vi "SP_Breakdown_Analysis.vi"() -> ()   [LabVIEW 2017]
uses:
  <vilib>/addons/database/Connection.llb/DB Tools Open Connec (Path).vi
  Globle/Login Data.vi
  <vilib>/addons/database/NI_Database_API.lvlib
panel:
  out "Elements Found out":string[](array[string])
  in  "Cancel Button - Archive":bool
  out "stackholder":string
  out "Role Id":string
  in  "Get Rport 2":bool
  in  "Download 2":bool
  out "Array":string[][](array[string])
  out "index of element":i32
  in  "Station":string(combo)
  out "error out":errorcluster
  in  "error in (no error)":errorcluster
  in  "Shift":string(combo)
  in  "Tab Control":enum32{"Statistical", "Graphical"}(tab)
  out "Table":string[][](table)
  out "Run-Time Status":cluster{dbl[], dbl[]}(graph)
  in  "To":timestamp format="%<%Y-%m-%d>T"
  in  "From":timestamp format="%<%Y-%m-%d>T"
  in  "Stakeholder":string(combo)
  # "Breakdown Analysis Report"
  # "Designed And Developed By - Infinity Automation Systems Pvt. Ltd."
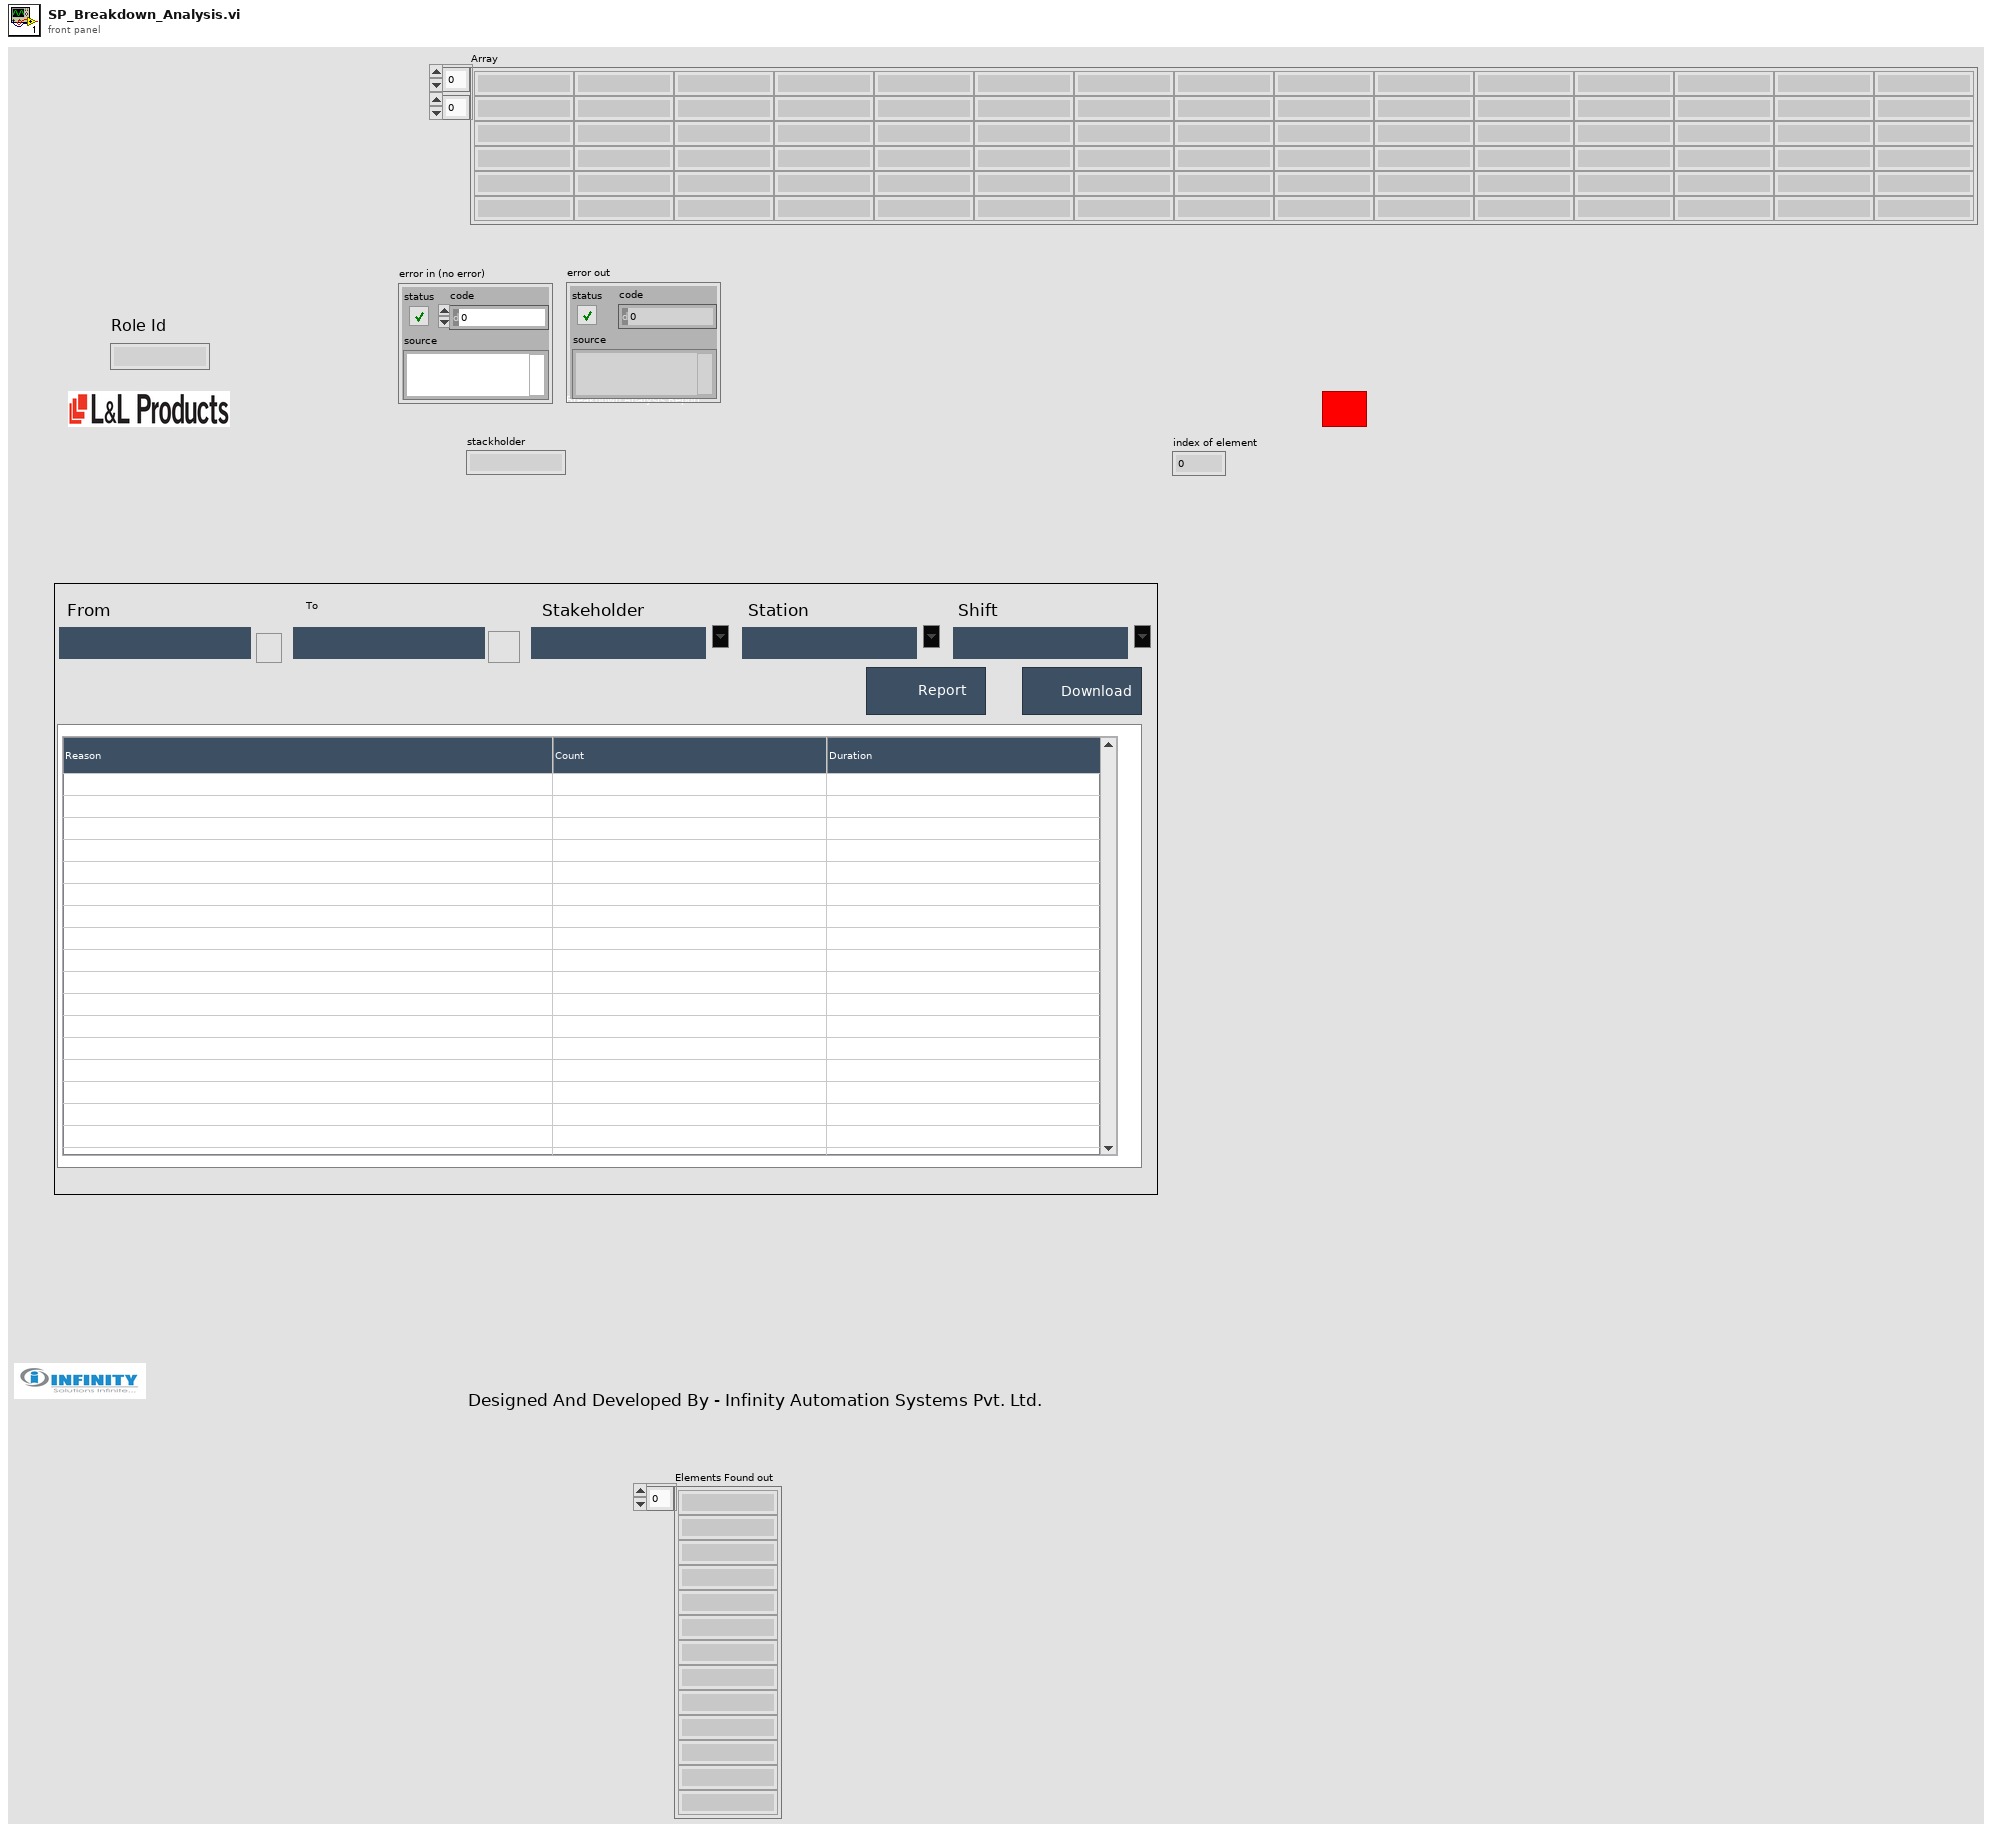
[diagram p1: front panel]
types:
  T1 = typedef "NI_Database_API.lvlib/Conn ObjectReference.ctl" = refnum<k1>
  T2 = enum32{"invalid app kind", "Development System", "Run Time System", "Student Edition", "Embedded LabVIEW", "Evaluation", "Custom"}
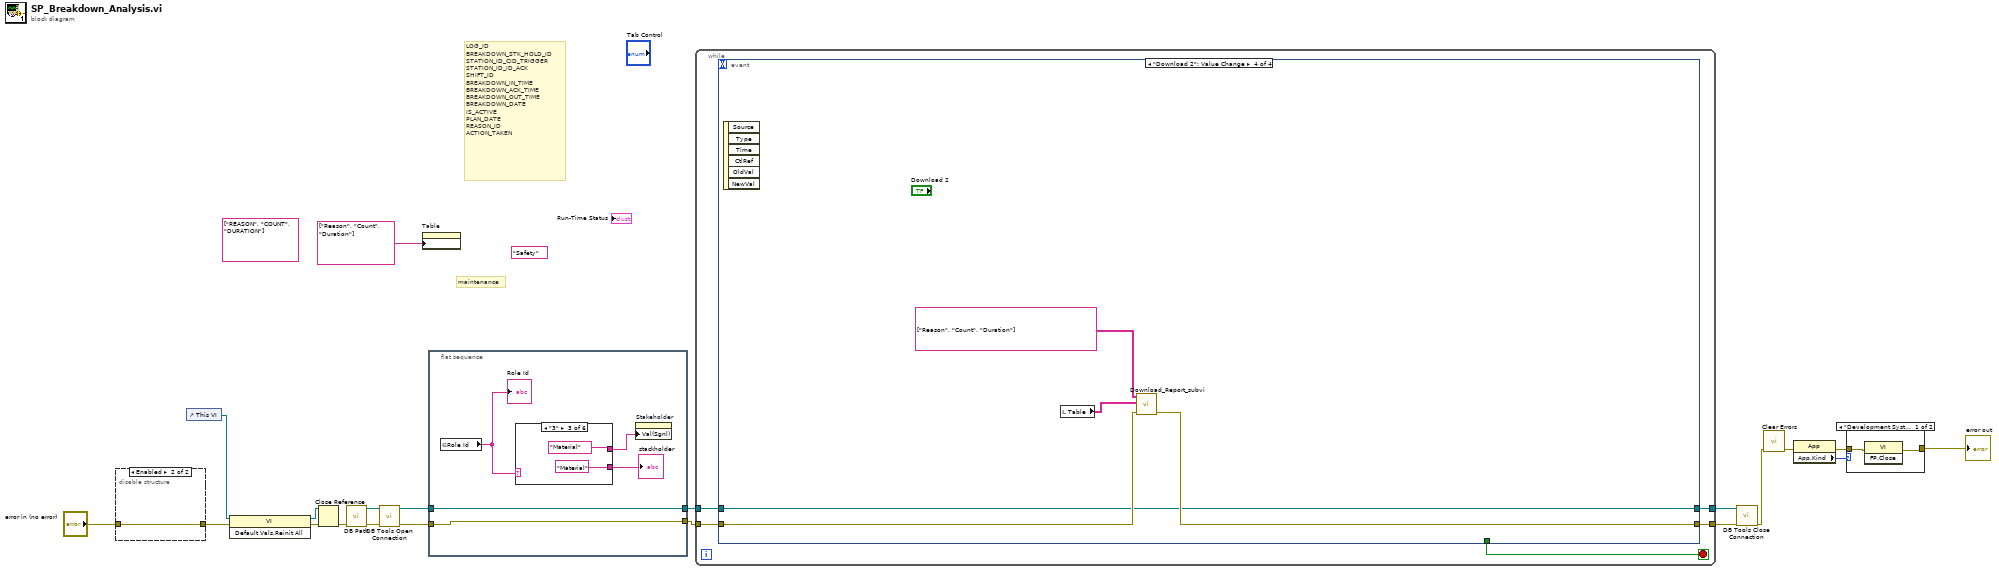
[diagram p0: block diagram]
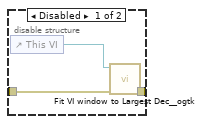
[diagram p2: hidden frame]
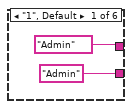
[diagram p3: hidden frame]
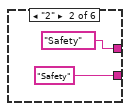
[diagram p4: hidden frame]
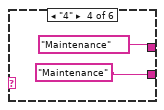
[diagram p5: hidden frame]
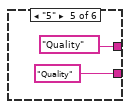
[diagram p6: hidden frame]
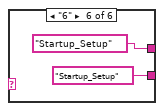
[diagram p7: hidden frame]
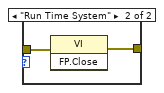
[diagram p8: hidden frame]
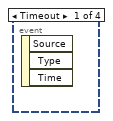
[diagram p9: hidden frame]
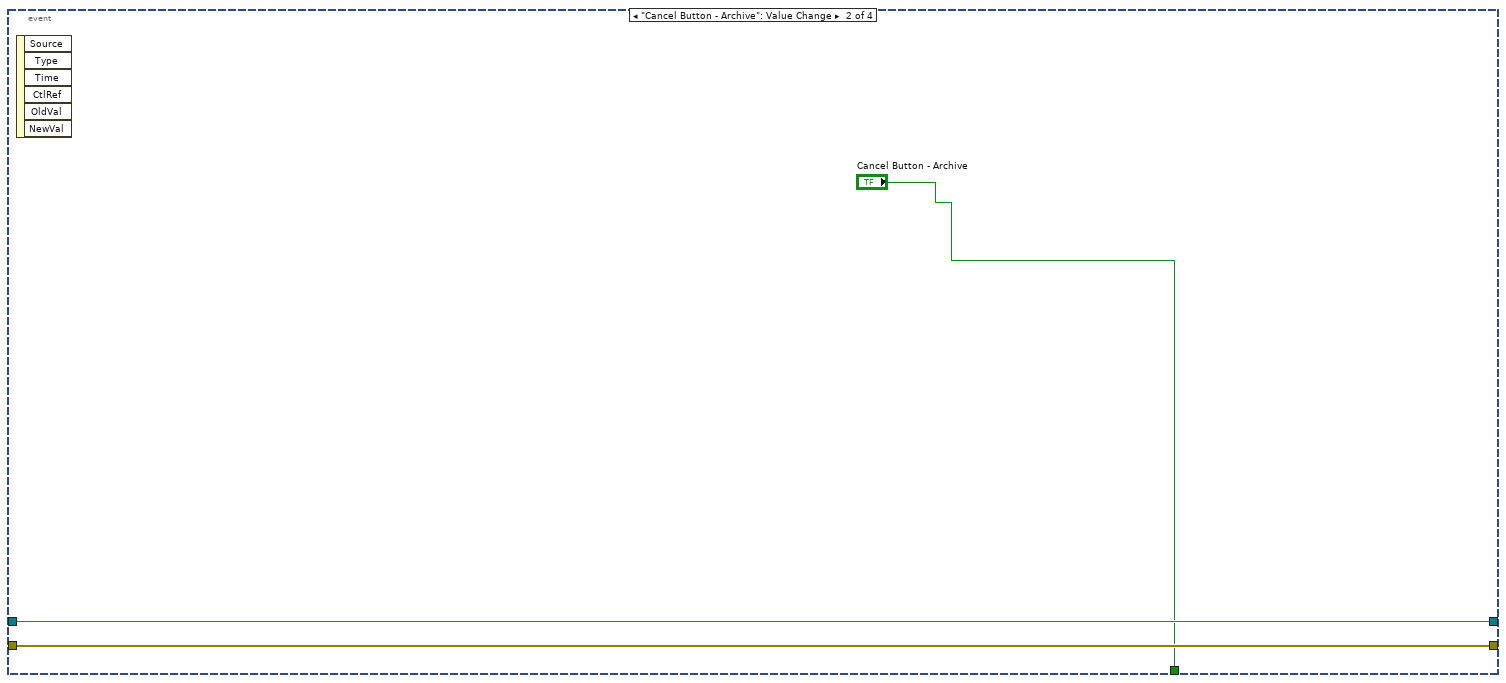
[diagram p10: hidden frame]
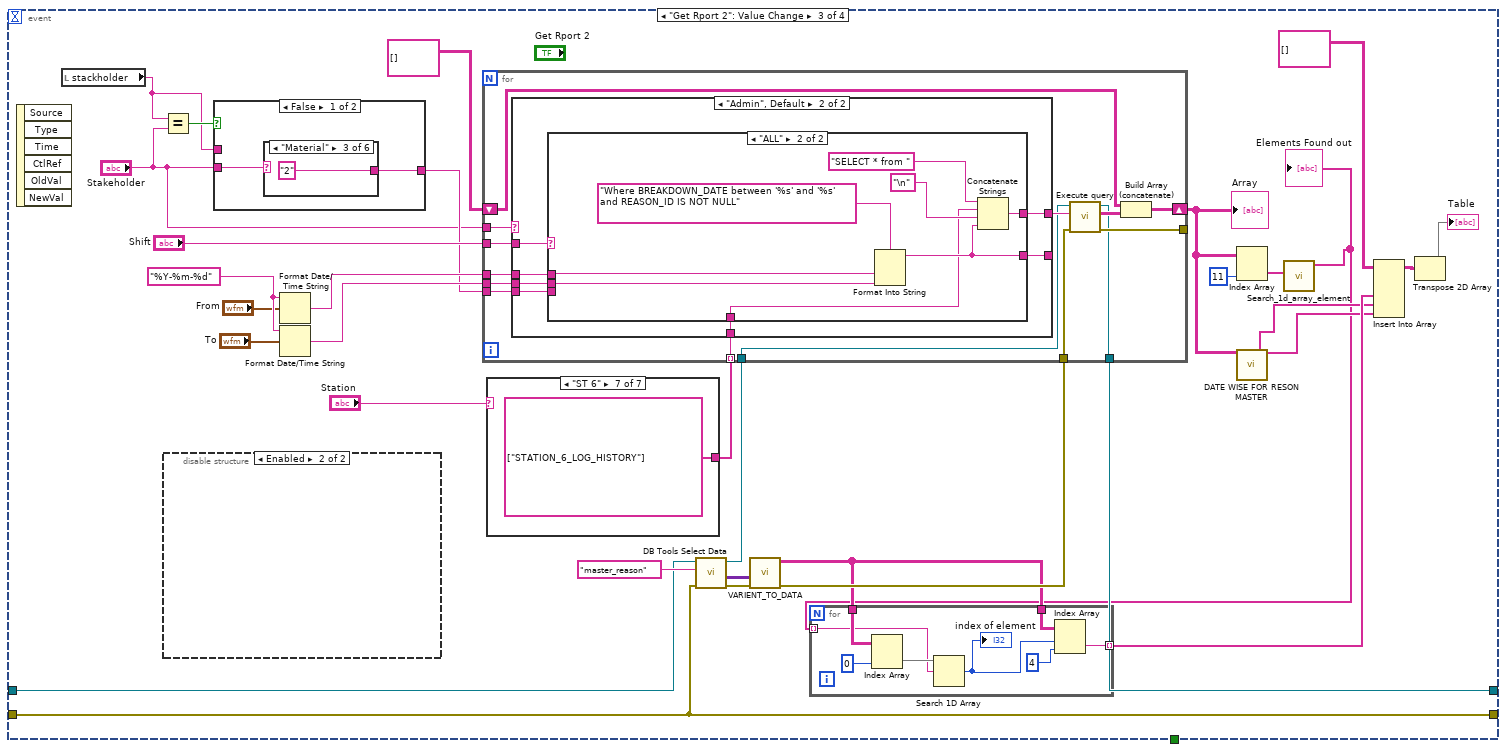
[diagram p11: hidden frame]
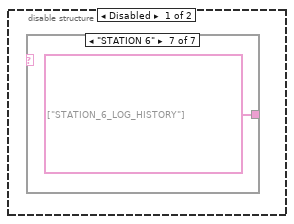
[diagram p12: hidden frame]
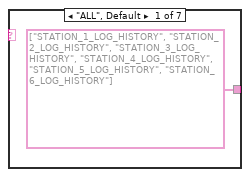
[diagram p13: hidden frame]
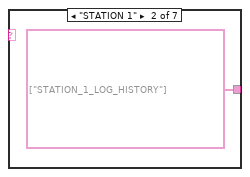
[diagram p14: hidden frame]
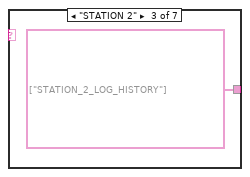
[diagram p15: hidden frame]
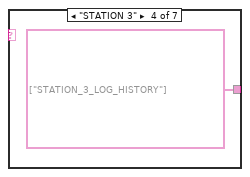
[diagram p16: hidden frame]
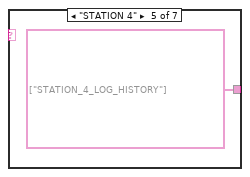
[diagram p17: hidden frame]
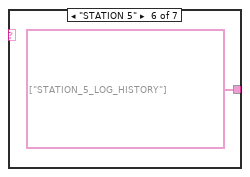
[diagram p18: hidden frame]
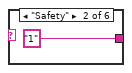
[diagram p20: hidden frame]
diagram:
  (unwired) string[] ["REASON", "COUNT", "DURATION"] ("Column Header Strings[]")
  (unwired) "Safety" ("Stakeholder")
  # "maintenance"
  # "LOG_ID\nBREAKDOWN_STK_HOLD_ID\nSTATION_ID_CID_TRIGGER\nSTATION_ID_ID_ACK\nSHIFT_ID\nBREAKDOWN_IN_TIME\nBREAKDOWN_ACK_TIME\nBREAKDOWN_OUT_TIME\nBREAKDOWN_DATE\nIS_ACTIVE\nPLAN_DATE\nREASON_ID\nACTION_TAKEN"
  n1 = disable-structure shown="Enabled" {
    disable-tunnel: "error in (no error)" -> [w23 w24]
    disable-tunnel: [w22 w24] -> w10
    frame Disabled {
      n2 = control-ref of="This VI"() -> (w21:refnum<vi>)
      n3 = call <userlib>:"Fit VI window to Largest Dec__ogtk.vi"("error in (no error)"=w23, "VI Ref (calling VI)"=w21) -> ("error out"=w22:errorcluster)  [unwired: 4 in, 1 out]
    }
    frame Enabled {
    }
  }
  n4 = control-ref of="This VI"() -> (w20:refnum<vi>)
  n5 = invoke class="VI" method="Default Vals.Reinit All"(reference=w20, error in=w10) -> (reference out=w18:refnum<vi>, error out=w19:errorcluster)  [unwired: 1 in, 1 out]
  n6 = Close Reference(reference=w18, error in (no error)=w19) -> (error out=w17:errorcluster)
  n7 = call "DB Path.vi"("error in"=w17) -> ("error out"=w16:errorcluster, "DB Path"=w15:path)  [unwired: 9 in]
  n8 = call-poly <vilib>:"DB Tools Open Connection.vi"("error in (no error)"=w16, "connection information"=w15) -> ("error out"=w3:errorcluster, "connection reference"=w1:T1)  [unwired: 6 in]
  n9 = property on="Table" class="Tbl (strict)"("Column Headers[]"=string[] ["Reason", "Count", "Duration"] ("Column Header Strings[]")) -> ()  [unwired: 2 in, 2 out]
  n10 = flat-sequence {
    tunnel: [w29] -> w4
    tunnel: w3 -> [w29]
    tunnel: [w28] -> w2
    tunnel: w1 -> [w28]
    frame #0 {
      n11 = global read "Login Data.vi" "Role Id"() -> (w25:string)
      "Role Id" <- w25
      n12 = case shown="\"3\"" w25 {
        tunnel: ["Admin" ("string") "Safety" "Material" "Maintenance" "Quality" "Startup_Setup"] -> w27
        tunnel: ["Admin" ("Stakeholder") "Safety" ("Stakeholder") "Material" ("Stakeholder") "Maintenance" ("Stakeholder") "Quality" ("Stakeholder") "Startup_Setup" ("Stakeholder")] -> w26
        frame "1", Default {
        }
        frame "2" {
        }
        frame "3" {
        }
        frame "4" {
        }
        frame "5" {
        }
        frame "6" {
        }
      }
      "stackholder" <- w27
      n13 = property on="Stakeholder" class="CmbBox"("Val(Sgnl)"=w26) -> ()  [unwired: 2 in, 2 out]
    }
  }
  n14 = while {
    tunnel: w4 -> [w45]
    tunnel: w2 -> [w44]
    tunnel: [w43] -> w12
    tunnel: [w42] -> w13
    stop <- w46 stop-if-true
    n15 = event shown="[3] \"Download 2\": Value Change" {
      selector: _ -> [_ _ _ _]
      dyn-events: _ -> [_ _ _ _]
      timeout: _ -> [_ _ _ _]
      tunnel: [_ "Cancel Button - Archive" _ _] -> w46
      tunnel: w45 -> [_ w49 w65 w179]
      tunnel: w44 -> [_ w48 w67 w177]
      tunnel: [_ w49 w65 w178] -> w43
      tunnel: [_ w48 w66 w177] -> w42
      event Timeout {
        n16 = event-data() -> ()  [unwired: 1 in, 3 out]
      }
      event "Cancel Button - Archive": Value Change {
        n17 = event-data() -> ()  [unwired: 1 in, 6 out]
      }
      event "Get Rport 2": Value Change {
        w80 = "%Y-%m-%d" ("time format string (%c)")
        n18 = event-data() -> ()  [unwired: 1 in, 6 out]
        n19 = local read "stackholder"() -> (w51:string)
        n20 = Equal?(x=w51, y="Stakeholder") -> (x = y?=w52:bool)
        n21 = disable-structure shown="Enabled" {
          frame Disabled {
            n22 = case shown="\"STATION 6\"" {
              selector: _ -> [_ _ _ _ _ _ _]
              tunnel: [string[] ["STATION_1_LOG_HISTORY", "STATION_2_LOG_HISTORY", "STATION_3_LOG_HISTORY", "STATION_4_LOG_HISTORY", "STATION_5_LOG_HISTORY", "STATION_6_LOG_HISTORY"] string[] ["STATION_1_LOG_HISTORY"] string[] ["STATION_2_LOG_HISTORY"] string[] ["STATION_3_LOG_HISTORY"] string[] ["STATION_4_LOG_HISTORY"] string[] ["STATION_5_LOG_HISTORY"] string[] ["STATION_6_LOG_HISTORY"]] -> _
              frame "ALL", Default {
              }
              frame "STATION 1" {
              }
              frame "STATION 2" {
              }
              frame "STATION 3" {
              }
              frame "STATION 4" {
              }
              frame "STATION 5" {
              }
              frame "STATION 6" {
              }
            }
          }
          frame Enabled {
          }
        }
        n23 = case shown="False" w52 {
          tunnel: [w90 _] -> w72
          tunnel: "Stakeholder" -> [w89 _]
          tunnel: w51 -> [_ _]
          frame False {
            n24 = case shown="\"Material\"" w89 {
              tunnel: [_ "1" "2" "3" "4" "5"] -> w90
              frame "Admin", Default {
              }
              frame "Safety" {
              }
              frame "Material" {
              }
              frame "Maintenance" {
              }
              frame "Quality" {
              }
              frame "Startup_Setup" {
              }
            }
          }
          frame True {
          }
        }
        n25 = Format Date/Time String(time format string (%c)=w80, seconds (now)="From") -> (date/time string=w77:string)  [unwired: 1 in]
        n26 = Format Date/Time String(time format string (%c)=w80, seconds (now)="To") -> (date/time string=w76:string)  [unwired: 1 in]
        n27 = case shown="\"ST 6\"" "Station" {
          tunnel: [string[] ["STATION_1_LOG_HISTORY", "STATION_2_LOG_HISTORY", "STATION_3_LOG_HISTORY", "STATION_4_LOG_HISTORY", "STATION_5_LOG_HISTORY", "STATION_6_LOG_HISTORY"] string[] ["STATION_1_LOG_HISTORY"] string[] ["STATION_2_LOG_HISTORY"] string[] ["STATION_3_LOG_HISTORY"] string[] ["STATION_4_LOG_HISTORY"] string[] ["STATION_5_LOG_HISTORY"] string[] ["STATION_6_LOG_HISTORY"]] -> w73
          frame "ALL", Default {
          }
          frame "ST 1" {
          }
          frame "ST 2" {
          }
          frame "ST 3" {
          }
          frame "ST 4" {
          }
          frame "ST 5" {
          }
          frame "ST 6" {
          }
        }
        n28 = call <vilib>:"DB Tools Select Data.vi"("error in (no error)"=w65, "table"="master_reason", "connection reference"=w67) -> ("error out"=w71:errorcluster, "data"=w70:variant[][], "connection reference out"=w68:T1)  [unwired: 3 in]
        n29 = call "VARIENT_TO_DATA.vi"("data"=w70, "error in (no error)"=w71) -> ("Table"=w63:string[][], "error out"=w64:errorcluster)  [unwired: 7 in]
        n30 = for {
          shift-right: [w122] -> w59
          shift-left: string[][] [] -> [w121]
          tunnel: [w120] -> _
          tunnel: [w119] -> w66
          tunnel: w77 -> [w118]
          tunnel: w76 -> [w117]
          tunnel: "Stakeholder" -> [w116]
          tunnel: "Shift" -> [w115]
          tunnel: w73 -> [w114] mode=indexing
          tunnel: w72 -> [w113]
          tunnel: w68 -> [w112]
          tunnel: w64 -> [w111]
          n31 = case shown="\"Admin\", Default" w116 {
            tunnel: [w131 w157] -> _
            tunnel: [w130 w156] -> w124
            tunnel: w118 -> [w129 w155]
            tunnel: w117 -> [w128 w154]
            tunnel: w115 -> [w127 w152]
            tunnel: w114 -> [w126 w151]
            tunnel: w113 -> [w125 w153]
            frame "False" {
              n32 = case shown="\"ALL\"" w127 {
                selector: w127 -> [w132 _]
                tunnel: [w137 w147] -> w131
                tunnel: [w138 w146] -> w130
                tunnel: w129 -> [w136 w144]
                tunnel: w128 -> [w135 w143]
                tunnel: w126 -> [w134 w145]
                tunnel: w125 -> [w133 w142]
                frame "False", Default {
                  n33 = Format Into String(format string="Where BREAKDOWN_DATE between '%s' and '%s' and BREAKDOWN_STK_HOLD_ID ='%s'  and SHIFT_ID='%s' and REASON_ID IS NOT NULL    " ("condition"), w136, w135, w133, w132) -> (resulting string=w137:string)  [unwired: 2 in, 1 out]
                  n34 = Concatenate Strings("SELECT * from " ("String"), w134, "\n" ("string"), w137) -> (w138:string)
                }
                frame "ALL" {
                  n35 = Format Into String(format string="Where BREAKDOWN_DATE between '%s' and '%s' and BREAKDOWN_STK_HOLD_ID ='%s' and REASON_ID IS NOT NULL" ("condition"), w144, w143, w142) -> (resulting string=w147:string)  [unwired: 2 in, 1 out]
                  n36 = Concatenate Strings("SELECT * from " ("String"), w145, "\n" ("string"), w147) -> (w146:string)
                }
              }
            }
            frame "Admin", Default {
              n37 = case shown="\"ALL\"" w152 {
                selector: w152 -> [w159 _]
                tunnel: [w162 w171] -> w157
                tunnel: [w163 w170] -> w156
                tunnel: w155 -> [w161 w168]
                tunnel: w154 -> [w160 w167]
                tunnel: w153 -> [_ _]
                tunnel: w151 -> [w158 w169]
                frame "False", Default {
                  n38 = Format Into String(format string="Where BREAKDOWN_DATE between '%s' and '%s' and SHIFT_ID='%s' and REASON_ID IS NOT NULL " ("condition"), w161, w160, w159) -> (resulting string=w162:string)  [unwired: 2 in, 1 out]
                  n39 = Concatenate Strings("SELECT * from " ("String"), w158, "\n" ("string"), w162) -> (w163:string)
                }
                frame "ALL" {
                  n40 = Format Into String(format string="Where BREAKDOWN_DATE between '%s' and '%s' and REASON_ID IS NOT NULL" ("condition"), w168, w167) -> (resulting string=w171:string)  [unwired: 2 in, 1 out]
                  n41 = Concatenate Strings("SELECT * from " ("String"), w169, "\n" ("string"), w171) -> (w170:string)
                }
              }
            }
          }
          n42 = call "Execute query.vi"("error in (no error)"=w111, "String"=w124, "connection reference"=w112) -> ("error out"=w120:errorcluster, "Table"=w123:string[][], "connection reference 2"=w119:T1)  [unwired: 5 in, 1 out]
          n43 = Build Array (concatenate)(w121, w123) -> (w122:string[][])
        }
        "Array" <- w59
        n44 = Index Array(array=w59, index (col)=11 ("disabled index (col)")) -> (element=w54:string[])  [unwired: 1 in]
        n45 = call "DATE WISE FOR RESON MASTER.vi"("Array"=w59) -> ("Count out"=w58:string[], "DURATION"=w57:string[])  [unwired: 12 in, 5 out]
        n46 = call "Search_1d_array_element.vi"("BD Date"=w54) -> ("Elements Found out"=w50:string[])  [unwired: 6 in, 2 out]
        "Elements Found out" <- w50
        n47 = for {
          tunnel: [w99] -> w61 mode=indexing
          tunnel: w63 -> [w98]
          tunnel: w63 -> [w97]
          tunnel: w50 -> [w96] mode=indexing
          n48 = Index Array(array=w98, index (col)=0 ("disabled index (col)")) -> (element=w102:string[])  [unwired: 1 in]
          n49 = Search 1D Array(1D array=w102, element=w96) -> (index of element=w103:i32)  [unwired: 1 in]
          "index of element" <- w103
          n50 = Index Array(array=w97, index (row)=w103, index (col)=4 ("disabled index (col)")) -> (element=w99:string)
        }
        n51 = Insert Into Array(array=string[][] [], new element #1=w61, new element #2=w58, new element #3=w57) -> (w56:string[][])  [unwired: 2 in]
        n52 = Transpose 2D Array(2D array=w56) -> (transposed array=→"Table":string[][])
      }
      event "Download 2": Value Change {
        n53 = event-data() -> ()  [unwired: 1 in, 6 out]
        n54 = local read "Table"() -> (w175:string[][])
        n55 = call "Download_Report_subvi.vi"("error in (no error)"=w179, "Value"=w175, "Column Header Strings[]"=string[][] [["Reason", "Count", "Duration"]]) -> ("error out"=w178:errorcluster)  [unwired: 8 in]
      }
    }
  }
  n56 = call <vilib>:"DB Tools Close Connection.vi"("error in (no error)"=w12, "connection reference"=w13) -> ("error out"=w6:errorcluster)  [unwired: 5 in]
  n57 = call <vilib>:"Clear Errors.vi"("error in (no error)"=w6) -> ("error out"=w9:errorcluster)  [unwired: 5 in, 1 out]
  n58 = property class="App"(error in=w9) -> (error out=w8:errorcluster, "App.Kind"=w7:T2)  [unwired: 1 in, 1 out]
  n59 = case shown="\"Development System\", Default" w7 {
    tunnel: w8 -> [w181 w183]
    tunnel: [w180 w182] -> w5
    frame "Development System", Default {
      n60 = invoke class="VI" method="FP.Close"(error in=w181) -> (error out=w180:errorcluster)  [unwired: 2 in, 2 out]
    }
    frame "Run Time System" {
      n61 = invoke class="VI" method="FP.Close"(error in=w183) -> (error out=w182:errorcluster)  [unwired: 2 in, 2 out]
    }
  }
  "error out" <- w5
